vi "Close Galil.vi"(6 "Disable?":bool, 7 "Command Input":string, 10 "error out 2":errorcluster, 11 "reference out 2":refnum<k7>) -> (2 "error out":errorcluster, 5 "Output String":string)   [LabVIEW 2011]
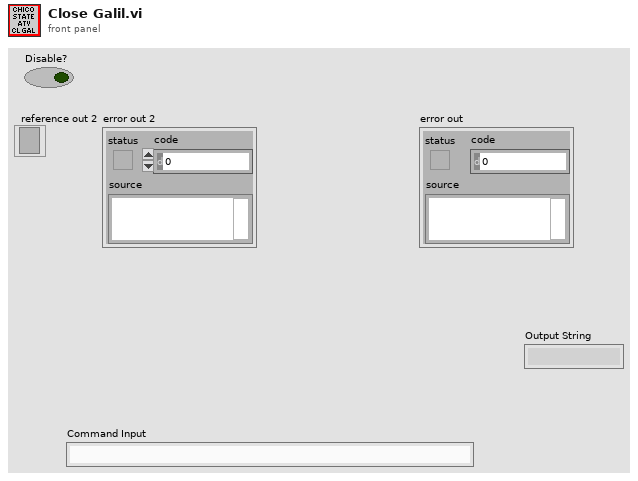
[diagram p1: front panel]
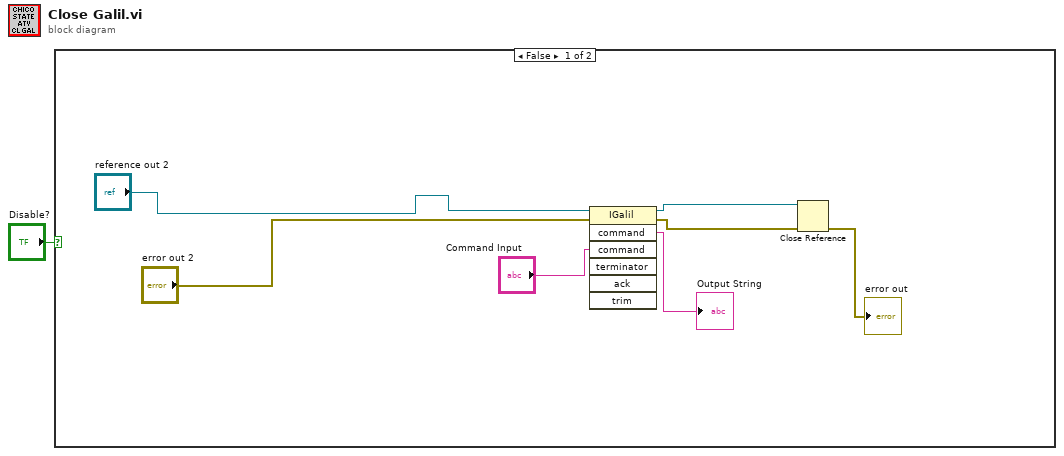
[diagram p0: block diagram]
diagram:
  n1 = case shown="False" "Disable?" {
    frame False {
      n2 = invoke class="IGalil" method="command"(reference="reference out 2", error in="error out 2", "command"="Command Input") -> (reference out=w4:refnum<k7>, error out=w3:errorcluster, "command"=→"Output String":string)  [unwired: 4 in, 4 out]
      n3 = Close Reference(reference=w4, error in (no error)=w3) -> (error out=→"error out":errorcluster)
    }
    frame True {
    }
  }
